vi "Protocol Settings.vi"(11 "Protocol":T2(ring)) -> (2 "Selected protocol":T2(ring), 3 "Protocol Settings":T1={"Frame Sync Edge for Channel 0"=enum."Falling", "Channel Count Per Frame"=2, "Channel Length"=32, "Bit Depth"=24, "Channel 0 Offset"=1, "Endianness"=enum."MSB First", "Data Justification"=enum."Left Justified", "Frame Length"=64, "Frame Sync Pulse Width"=32, "Bit Clock Edge  Sync"=enum."Falling"})   [LabVIEW 2021]
uses:
  C:/Program Files/National Instruments/LabVIEW 2021/examples/Digital Audio Acquisition and Generation Toolkit/subVIs/PCM Interface Type.ctl
  <vilib>/PDM Acquisition Toolkit/shared/controls/Digital Edge.ctl
  <vilib>/PDM Acquisition Toolkit/shared/PDM Shared.lvlib
panel:
  in  "Bit Clock Edge  Sync":enum8{"Rising", "Falling"}(ring)=enum."Falling"
  in  "Frame Sync Pulse Width":u16=32
  in  "Frame Length":u16=64
  in  "Data Justification":enum16{"Left Justified", "Right Justified"}(ring)
  in  "Endianness":enum16{"MSB First", "LSB First"}(ring)
  in  "Channel 0 Offset":u16=1
  in  "Bit Depth":u8=24
  in  "Channel Length":u16=32
  in  "Channel Count Per Frame":u8=2
  in  "Frame Sync Edge for Channel 0":enum16{"Rising", "Falling"}(ring)=enum."Falling"
  # "PCM data configuration"
  # "Frame sync clock control"
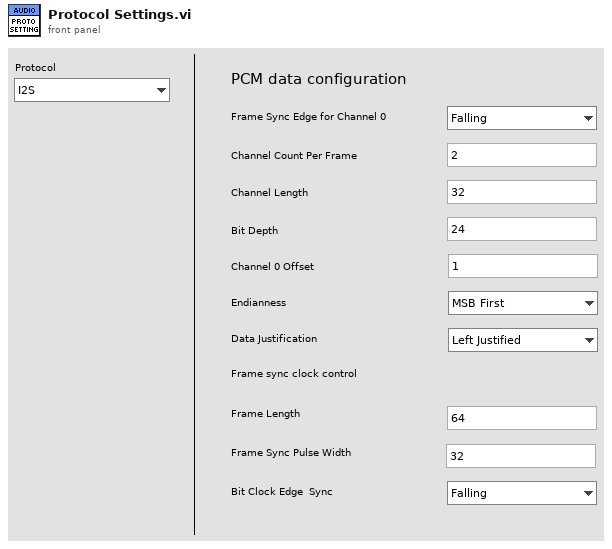
[diagram p1: front panel]
types:
  T1 = cluster{"Frame Sync Edge for Channel 0":enum16{"Rising", "Falling"}, "Channel Count Per Frame":u8, "Channel Length":u16, "Bit Depth":u8, "Channel 0 Offset":u16, "Endianness":enum16{"MSB First", "LSB First"}, "Data Justification":enum16{"Left Justified", "Right Justified"}, "Frame Length":u16, "Frame Sync Pulse Width":u16, "Bit Clock Edge  Sync":enum8{"Rising", "Falling"}}
  T2 = enum16{"I2S", "Left Justified", "Right Justified", "TDM"}
  T3 = enum32{"Invalid", "Standard", "Closed", "Hidden", "Minimized", "Maximized"}
  T4 = typedef "PDM Shared.lvlib/Digital Edge.ctl" = enum8{"Rising", "Falling"}
  T5 = typedef "PCM Interface Type.ctl" = enum16{"I2S", "Left Justified", "Right Justified", "TDM 4 Channel", "TDM 6 Channel", "TDM 8 Channel", "DSP mode", "DSP mode with 1 bit delay", "PCM Short Frame", "PCM Long Frame"}
  T6 = typedef "PDM Shared.lvlib/PCM Frame Sync Control.ctl" = cluster{"Frame Length":u16, "Frame Sync Pulse Width":u16, "Bit Clock Edge  Sync":T4}
  T7 = typedef "PDM Shared.lvlib/PCM Data Format Configuration.ctl" = cluster{"Frame Sync Edge for Channel 0":T4, "Channel Count Per Frame":u8, "Channel Length":u16, "Bit Depth":u8, "Channel 0 Offset":u16, "Endianness":T8, "Data Justification":T9}
  T8 = typedef "PDM Shared.lvlib/PCM Bit Endianness.ctl" = enum16{"MSB First", "LSB First"}
  T9 = typedef "PDM Shared.lvlib/PCM Data Justification.ctl" = enum16{"Left Justified", "Right Justified"}
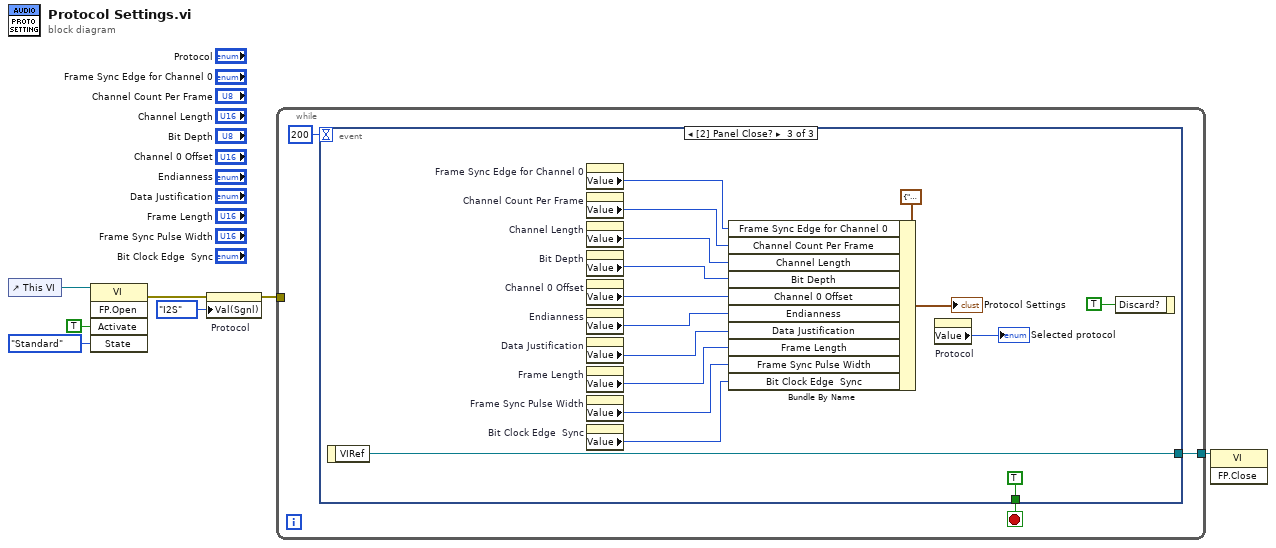
[diagram p0: block diagram]
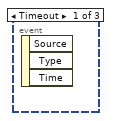
[diagram p2: hidden frame]
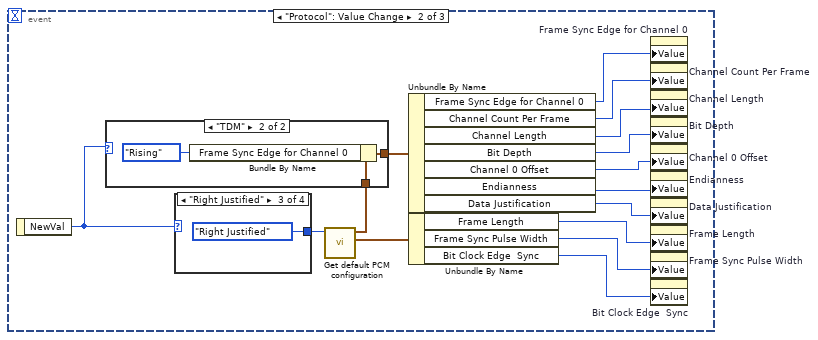
[diagram p3: hidden frame]
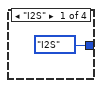
[diagram p5: hidden frame]
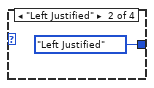
[diagram p6: hidden frame]
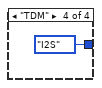
[diagram p7: hidden frame]
diagram:
  n1 = control-ref of="This VI"() -> (w5:refnum<vi>)
  n2 = invoke class="VI" method="FP.Open"(reference=w5, "Activate"=TRUE ("Activate?"), "State"=T3."Standard") -> (error out=w4:errorcluster)  [unwired: 2 in, 4 out]
  n3 = property on="Protocol" class="Enum (strict)"(error in=w4, "Val(Sgnl)"=T2."I2S" ("Value (Signaling)")) -> (error out=w3:errorcluster)  [unwired: 1 in, 1 out]
  n4 = while {
    tunnel: [w8] -> w1
    tunnel: w3 -> [_]
    stop <- w10 stop-if-true
    n5 = event shown="[2] Panel Close?" {
      selector: _ -> [_ _ _]
      dyn-events: _ -> [_ _ _]
      timeout: 200 -> [_ _ _]
      tunnel: [_ _ TRUE] -> w10
      tunnel: [_ _ w35] -> w8
      event Timeout {
        n6 = event-data() -> ()  [unwired: 1 in, 3 out]
      }
      event "Protocol": Value Change {
        n7 = event-data() -> ("NewVal"=w11:T2)  [unwired: 1 in]
        n8 = case shown="\"Right Justified\"" w11 {
          tunnel: [PCM_Interface_Type."I2S" ("PCM Interfaces") PCM_Interface_Type."Left Justified" ("PCM Interfaces") PCM_Interface_Type."Right Justified" ("PCM Interfaces") PCM_Interface_Type."I2S" ("PCM Interfaces")] -> w14
          frame "I2S" {
          }
          frame "Left Justified" {
          }
          frame "Right Justified" {
          }
          frame "TDM" {
          }
        }
        n9 = call "Get default PCM configuration.vi"("PCM Interfaces"=w14) -> ("Frame Sync Clock Control"=w13:T6, "PCM Data Configuration"=w15:T7)  [unwired: 9 in]
        n10 = case shown="\"TDM\"" w11 {
          tunnel: w15 -> [w26 w29]
          tunnel: [w26 w27] -> w12
          frame "I2S", Default {
          }
          frame "TDM" {
            n11 = Bundle By Name(cluster=w29, "Frame Sync Edge for Channel 0"=Digital_Edge."Rising") -> (w27:T7)
          }
        }
        n12 = Unbundle By Name(w12) -> ("Frame Sync Edge for Channel 0"=w25:T4, "Channel Count Per Frame"=w24:u8, "Channel Length"=w23:u16, "Bit Depth"=w22:u8, "Channel 0 Offset"=w21:u16, "Endianness"=w20:T8, "Data Justification"=w19:T9)
        n13 = Unbundle By Name(w13) -> ("Frame Length"=w18:u16, "Frame Sync Pulse Width"=w17:u16, "Bit Clock Edge  Sync"=w16:T4)
        n14 = property on="Frame Sync Edge for Channel 0" class="Enum (strict)"("Value"=w25) -> ()  [unwired: 2 in, 2 out]
        n15 = property on="Channel Count Per Frame" class="DigNum (strict)"("Value"=w24) -> ()  [unwired: 2 in, 2 out]
        n16 = property on="Channel Length" class="DigNum (strict)"("Value"=w23) -> ()  [unwired: 2 in, 2 out]
        n17 = property on="Bit Depth" class="DigNum (strict)"("Value"=w22) -> ()  [unwired: 2 in, 2 out]
        n18 = property on="Channel 0 Offset" class="DigNum (strict)"("Value"=w21) -> ()  [unwired: 2 in, 2 out]
        n19 = property on="Endianness" class="Enum (strict)"("Value"=w20) -> ()  [unwired: 2 in, 2 out]
        n20 = property on="Data Justification" class="Enum (strict)"("Value"=w19) -> ()  [unwired: 2 in, 2 out]
        n21 = property on="Frame Length" class="DigNum (strict)"("Value"=w18) -> ()  [unwired: 2 in, 2 out]
        n22 = property on="Frame Sync Pulse Width" class="DigNum (strict)"("Value"=w17) -> ()  [unwired: 2 in, 2 out]
        n23 = property on="Bit Clock Edge  Sync" class="Enum (strict)"("Value"=w16) -> ()  [unwired: 2 in, 2 out]
      }
      event Panel Close? {
        n24 = event-data() -> ("VIRef"=w35:refnum<vi>)  [unwired: 1 in]
        n25 = property on="Frame Sync Edge for Channel 0" class="Enum (strict)"() -> ("Value"=w47:enum16{"Rising", "Falling"})  [unwired: 2 in, 2 out]
        n26 = property on="Channel Count Per Frame" class="DigNum (strict)"() -> ("Value"=w46:u8)  [unwired: 2 in, 2 out]
        n27 = property on="Channel Length" class="DigNum (strict)"() -> ("Value"=w45:u16)  [unwired: 2 in, 2 out]
        n28 = property on="Bit Depth" class="DigNum (strict)"() -> ("Value"=w44:u8)  [unwired: 2 in, 2 out]
        n29 = property on="Channel 0 Offset" class="DigNum (strict)"() -> ("Value"=w36:u16)  [unwired: 2 in, 2 out]
        n30 = property on="Endianness" class="Enum (strict)"() -> ("Value"=w43:enum16{"MSB First", "LSB First"})  [unwired: 2 in, 2 out]
        n31 = property on="Data Justification" class="Enum (strict)"() -> ("Value"=w37:enum16{"Left Justified", "Right Justified"})  [unwired: 2 in, 2 out]
        n32 = property on="Frame Length" class="DigNum (strict)"() -> ("Value"=w42:u16)  [unwired: 2 in, 2 out]
        n33 = property on="Frame Sync Pulse Width" class="DigNum (strict)"() -> ("Value"=w41:u16)  [unwired: 2 in, 2 out]
        n34 = property on="Bit Clock Edge  Sync" class="Enum (strict)"() -> ("Value"=w40:enum8{"Rising", "Falling"})  [unwired: 2 in, 2 out]
        n35 = Bundle By Name(cluster=T1 {"Frame Sync Edge for Channel 0"=enum."Falling", "Channel Count Per Frame"=2, "Channel Length"=32, "Bit Depth"=24, "Channel 0 Offset"=1, "Endianness"=enum."MSB First", "Data Justification"=enum."Left Justified", "Frame Length"=64, "Frame Sync Pulse Width"=32, "Bit Clock Edge  Sync"=enum."Falling"} ("Protocol Settings"), "Frame Sync Edge for Channel 0"=w47, "Channel Count Per Frame"=w46, "Channel Length"=w45, "Bit Depth"=w44, "Channel 0 Offset"=w36, "Endianness"=w43, "Data Justification"=w37, "Frame Length"=w42, "Frame Sync Pulse Width"=w41, "Bit Clock Edge  Sync"=w40) -> (→"Protocol Settings":T1)
        n36 = property on="Protocol" class="Enum (strict)"() -> ("Value"=→"Selected protocol":T2)  [unwired: 2 in, 2 out]
        n37 = event-data("Discard?"=TRUE) -> ()  [unwired: 1 in, 1 out]
      }
    }
  }
  n38 = invoke class="VI" method="FP.Close"(reference=w1) -> ()  [unwired: 2 in, 3 out]
